vi "CreateNewWizard_IncludeItem.vi"(11 "Wizard":T1) -> (3 "Include me":bool)   [LabVIEW 2023, in "Add Async Methods Actor.lvlib"]
uses:
  Add Async Methods Actor.lvlib
  <resource>/Framework/Providers/API/ItemRef.ctl
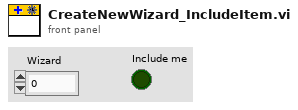
[diagram p1: front panel]
types:
  T1 = typedef "ItemRef.ctl" = u64
  T2 = typedef "mxLvNIIM.ctl" = cluster{"Item URL":string, "Item ID":string, "Item Index":i32, "Specific Type":string}
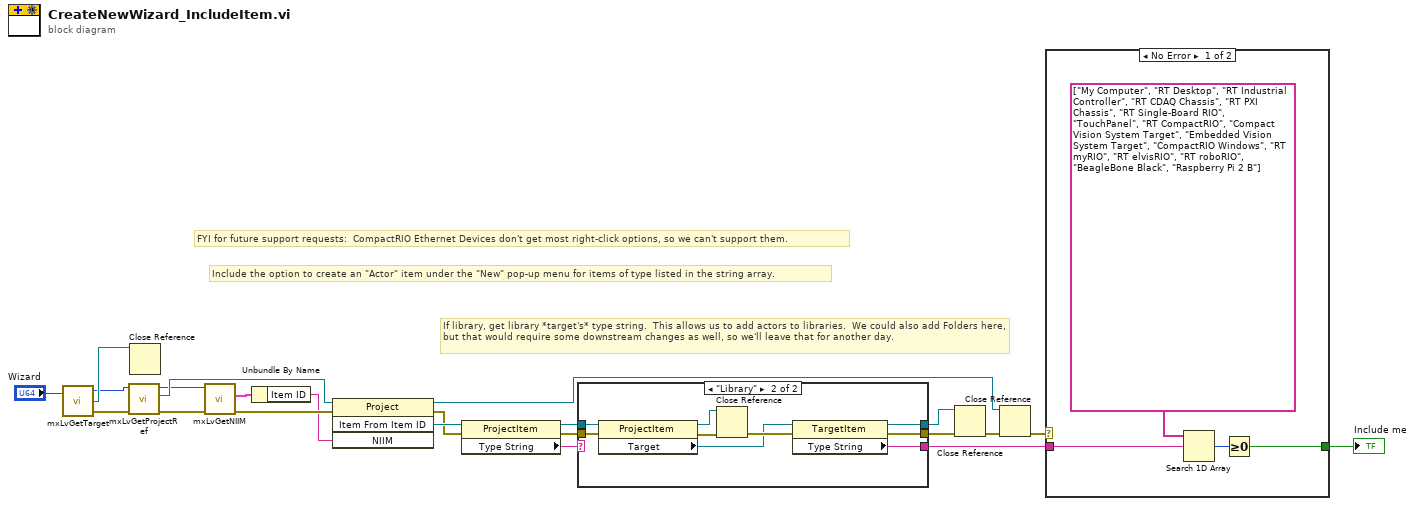
[diagram p0: block diagram]
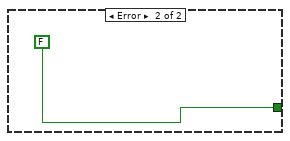
[diagram p3: hidden frame]
diagram:
  # "FYI for future support requests:  CompactRIO Ethernet Devices don't get most right-click options, so we can't support them."
  # "If library, get library *target's* type string.  This allows us to add actors to libraries.  We could also add Folders here, but that would require some downstream changes as well, so we'll leave that for another day."
  # "Include the option to create an \"Actor\" item under the \"New\" pop-up menu for items of type listed in the string array."
  n1 = call <resource>:"mxLvGetTarget.vi"("Item"="Wizard") -> ("Item"=w14:T1, "Target"=w16:refnum<vi>, "error out"=w15:errorcluster)  [unwired: 1 in]
  n2 = call <resource>:"mxLvGetProjectRef.vi"("error in"=w15, "Item"=w14) -> ("error out"=w21:errorcluster, "Project Refnum"=w17:refnum<vi>, "Item"=w12:T1)  [unwired: 7 in]
  n3 = Close Reference(reference=w16) -> ()  [unwired: 1 in, 1 out]
  n4 = call <resource>:"mxLvGetNIIM.vi"("error in"=w21, "Item"=w12) -> ("error out"=w19:errorcluster, "NIIM"=w18:T2)  [unwired: 7 in, 1 out]
  n5 = Unbundle By Name(w18) -> ("Item ID"=w1:string)
  n6 = invoke class="Project" method="Item From Item ID"(reference=w17, error in=w19, "NIIM"=w1) -> (reference out=w4:refnum<vi>, error out=w9:errorcluster, "GetItemFromNIIM"=w20:refnum<vi>)  [unwired: 1 in, 1 out]
  n7 = property class="ProjectItem"(reference=w20, error in=w9) -> (reference out=w10:refnum<vi>, error out=w11:errorcluster, "Type String"=w3:string)
  n8 = case shown="\"Library\"" w3 {
    selector: w3 -> [w23 _]
    tunnel: w11 -> [w24 w33]
    tunnel: w10 -> [w25 w34]
    tunnel: [w23 w32] -> w2
    tunnel: [w24 w31] -> w8
    tunnel: [w25 w30] -> w7
    frame Default {
    }
    frame "Library" {
      n9 = property class="ProjectItem"(reference=w34, error in=w33) -> (reference out=w28:refnum<vi>, error out=w29:errorcluster, "Target"=w26:refnum<vi>)
      n10 = Close Reference(reference=w28, error in (no error)=w29) -> (error out=w27:errorcluster)
      n11 = property class="TargetItem"(reference=w26, error in=w27) -> (reference out=w30:refnum<vi>, error out=w31:errorcluster, "Type String"=w32:string)
    }
  }
  n12 = Close Reference(reference=w7, error in (no error)=w8) -> (error out=w6:errorcluster)
  n13 = Close Reference(reference=w4, error in (no error)=w6) -> (error out=w5:errorcluster)
  n14 = case shown="No Error" w5 {
    tunnel: w2 -> [w38 _]
    tunnel: [w36 FALSE] -> w22
    frame No Error {
      n15 = Search 1D Array(1D array=string[] ["My Computer", "RT Desktop", "RT Industrial Controller", "RT CDAQ Chassis", "RT PXI Chassis", "RT Single-Board RIO", "TouchPanel", "RT CompactRIO", "Compact Vision System Target", "Embedded Vision System Target", "CompactRIO Windows", "RT myRIO", "RT elvisRIO", "RT roboRIO", "BeagleBone Black", "Raspberry Pi 2 B"] ("Array"), element=w38) -> (index of element=w37:i32)  [unwired: 1 in]
      n16 = Greater Or Equal To 0?(x=w37) -> (x >= 0?=w36:bool)
    }
    frame Error {
    }
  }
  "Include me" <- w22
